vi "6733_write_waveform.vi"(8 "Error In":errorcluster, 9 "Control Task In":refnum<k21>, 10 "Waveform Task In":refnum<k21>, 11 "Inputs":T1 {"Waveform Parameters"."Degree (polynomial only)" min=1}) -> (0 "error out":errorcluster, 2 "counter task out":refnum<k21>, 3 "waveform task out":refnum<k21>)   [LabVIEW 2013]
uses:
  Control 1.ctl
  <vilib>/DAQmx/write.llb/DAQmx Write (Analog 1D DBL NChan 1Samp).vi
  <vilib>/DAQmx/write.llb/DAQmx Write (Analog 1D Wfm NChan NSamp).vi
  <vilib>/DAQmx/create/channels.llb/DAQmx Create Channel (AO-Voltage-Basic).vi
  <vilib>/DAQmx/miscellaneous.llb/DAQmx Fill In Error Info.vi
  <vilib>/Waveform/WDTOps.llb/WDT Append Waveforms DBL.vi
  <vilib>/DAQmx/configure/timing.llb/DAQmx Timing (Sample Clock).vi
  <vilib>/DAQmx/create/channels.llb/DAQmx Create Channel (CO-Pulse Generation-Frequency).vi
  <vilib>/DAQmx/configure/timing.llb/DAQmx Timing (Implicit).vi
  <vilib>/DAQmx/configure/trigger.llb/DAQmx Start Trigger (Digital Edge).vi
  <vilib>/Waveform/WDTOps.llb/WDT Scale Delta t DBL.vi
  <resource>/objmgr/daqmx.rc
panel:
  out "Total Time":dbl
  out "Sample Rate":dbl
  out "element":waveform(dbl)(graph)
  in  "index":i32
  out "Waveforms":waveform(dbl)[](array[waveform])
  out "Max Sample Rate":dbl=1000000.0
  out "# Inactive Channels":i32
  out "# Active Channels":i16
  out "Inactive Channels":tag[](array[tag])
  out "Active Channels":tag[](array[tag])
  out "Samples Written":dbl
  out "Voltage Maximum":dbl
  out "Voltage Minimum":dbl
  out "AO.PhysicalChans":tag[](array[tag])
  out "Active Device":tag
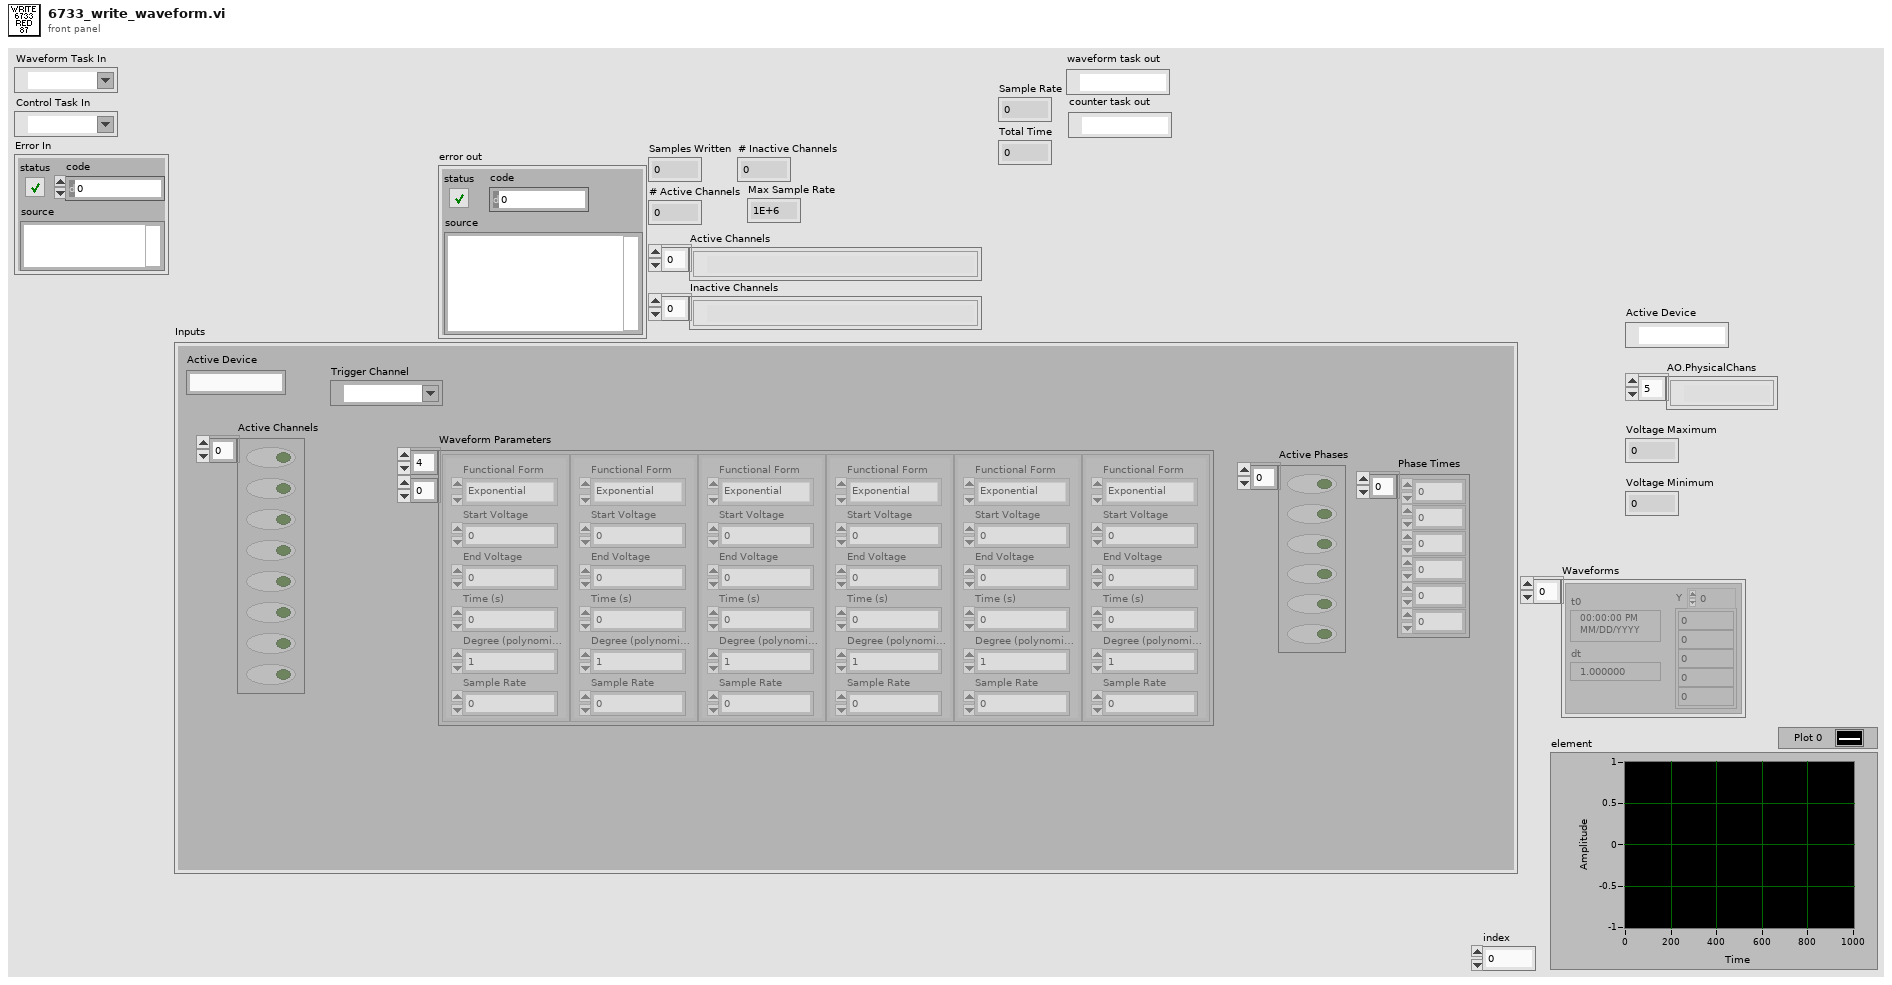
[diagram p1: front panel]
types:
  T1 = cluster{"Active Device":string, "Active Channels":bool[], "Waveform Parameters":cluster{"Functional Form":enum16{"Polynomial", "Exponential"}, "Start Voltage":dbl, "End Voltage":dbl, "Time (s)":dbl, "Degree (polynomial only)":i8, "Sample Rate":dbl}[][], "Active Phases":bool[], "Phase Times":dbl[], "Trigger Channel":tag}
  T2 = typedef "Control 1.ctl" = enum16{"Initialize", "Get Device Information", "Get Active/Inactive Channels", "Maximize Samples / Channel", "Write Waveforms", "Check for Problems", "Clear Old Tasks", "Write to cards"}
  T3 = cluster{"Functional Form":enum16{"Polynomial", "Exponential"}, "Start Voltage":dbl, "End Voltage":dbl, "Time (s)":dbl, "Degree (polynomial only)":i8, "Sample Rate":dbl}[][]
  T4 = cluster{"Functional Form":enum16{"Polynomial", "Exponential"}, "Start Voltage":dbl, "End Voltage":dbl, "Time (s)":dbl, "Degree (polynomial only)":i8, "Sample Rate":dbl}[]
  T5 = cluster{"Functional Form":enum16{"Polynomial", "Exponential"}, "Start Voltage":dbl, "End Voltage":dbl, "Time (s)":dbl, "Degree (polynomial only)":i8, "Sample Rate":dbl}
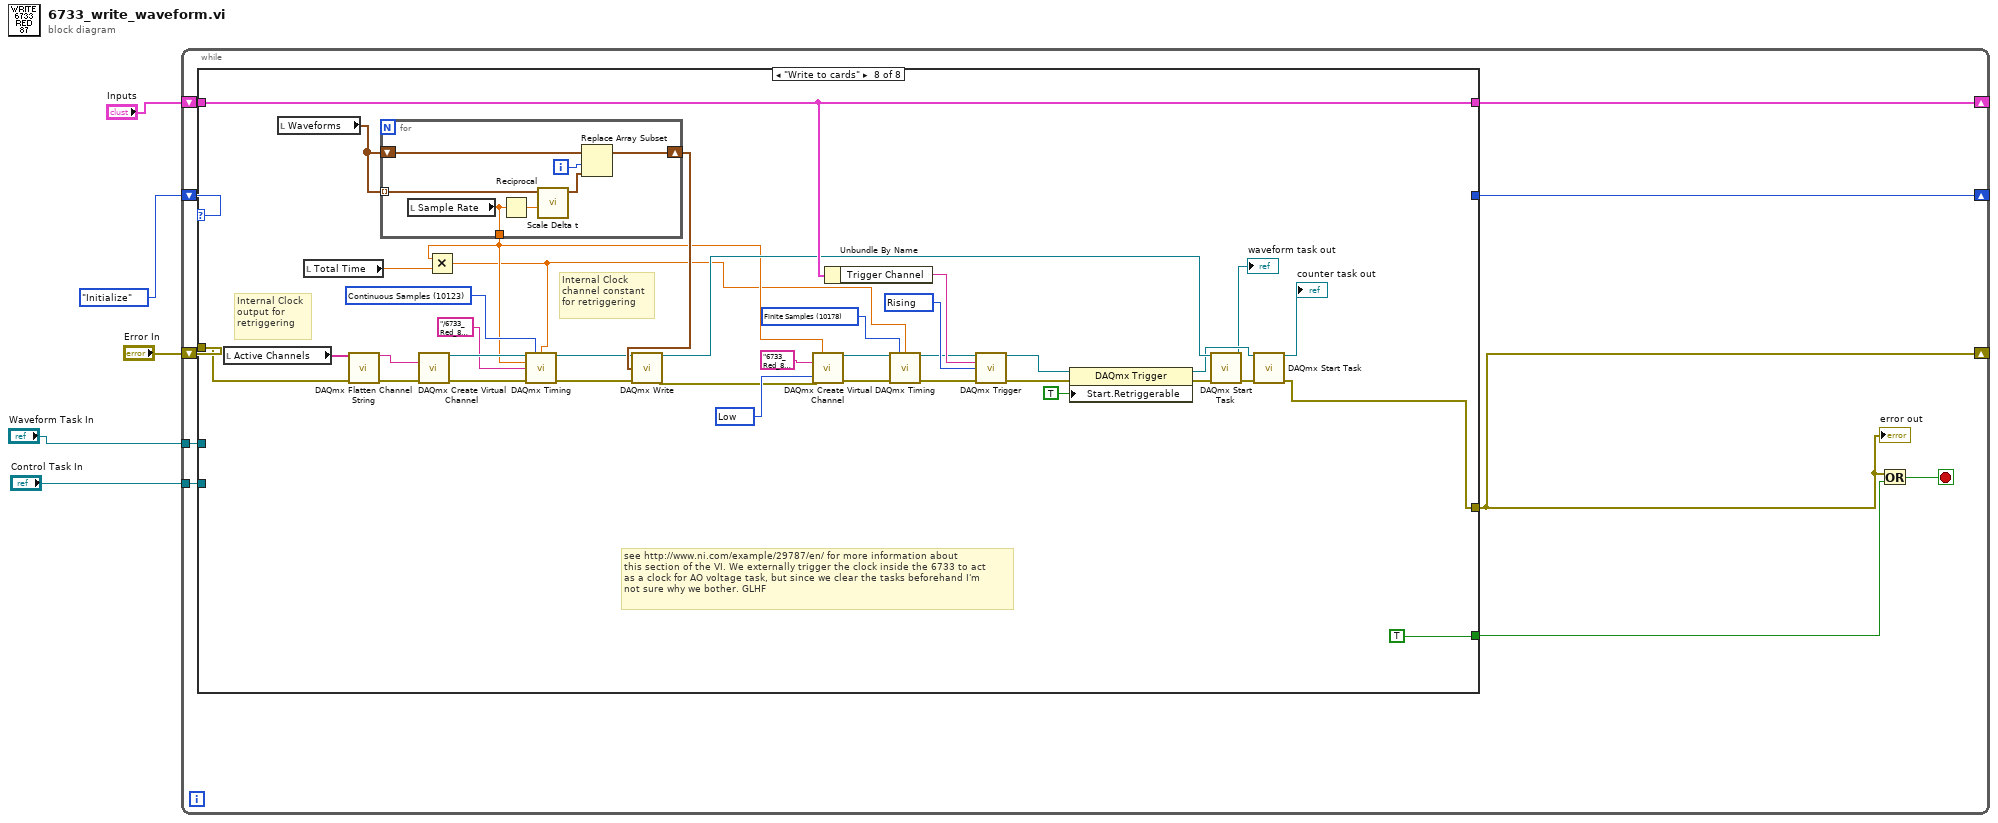
[diagram p0: block diagram]
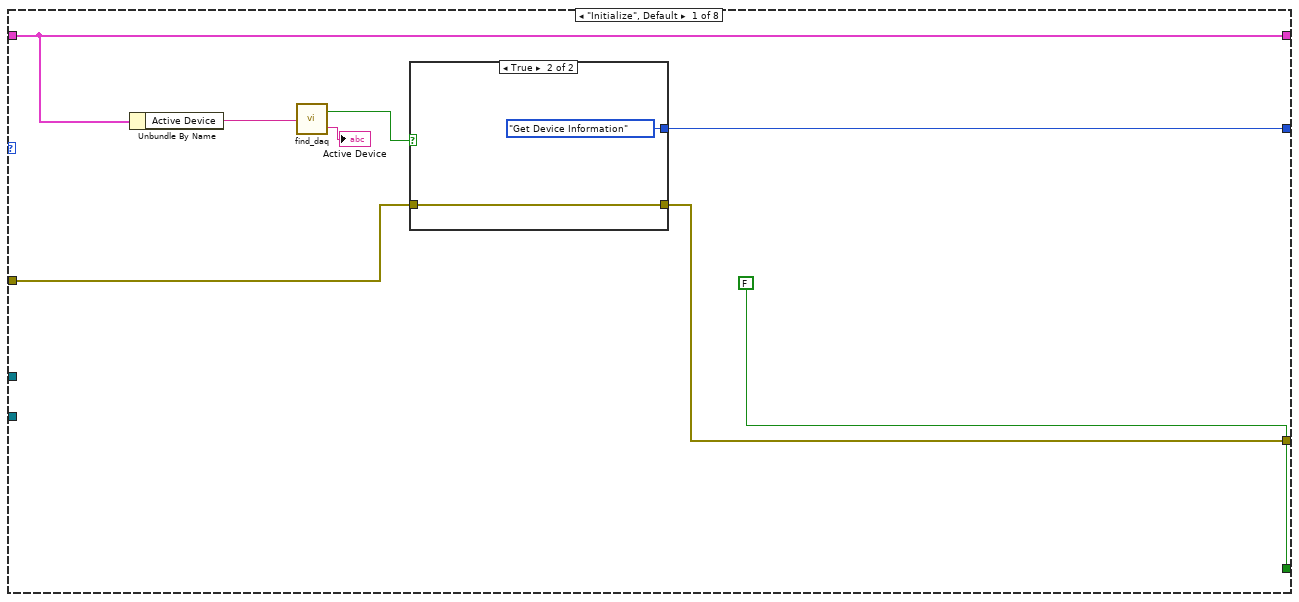
[diagram p2: hidden frame]
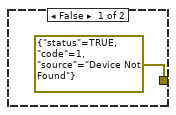
[diagram p3: hidden frame]
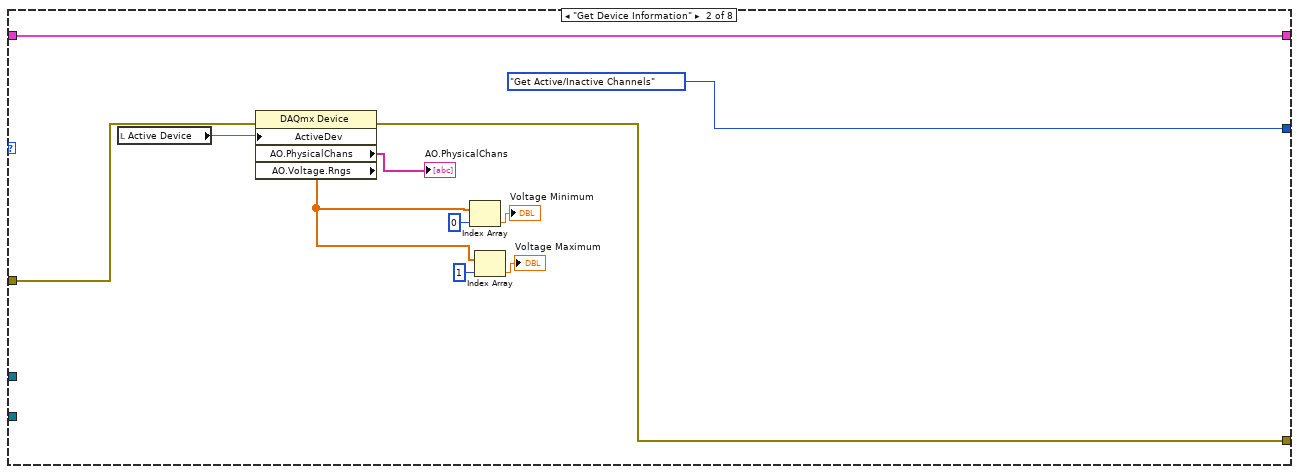
[diagram p4: hidden frame]
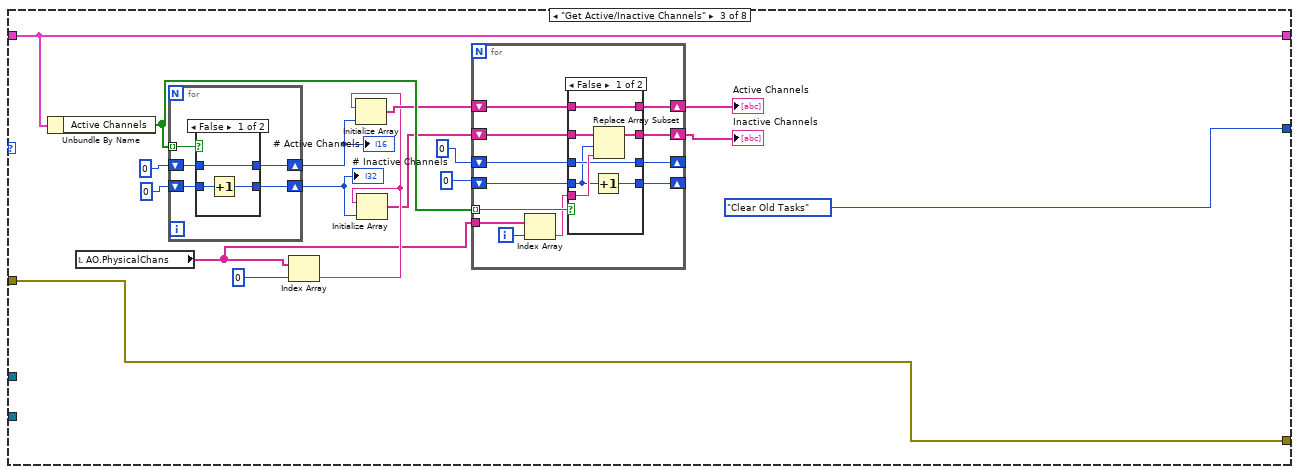
[diagram p5: hidden frame]
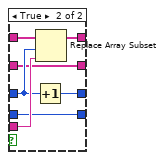
[diagram p6: hidden frame]
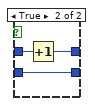
[diagram p7: hidden frame]
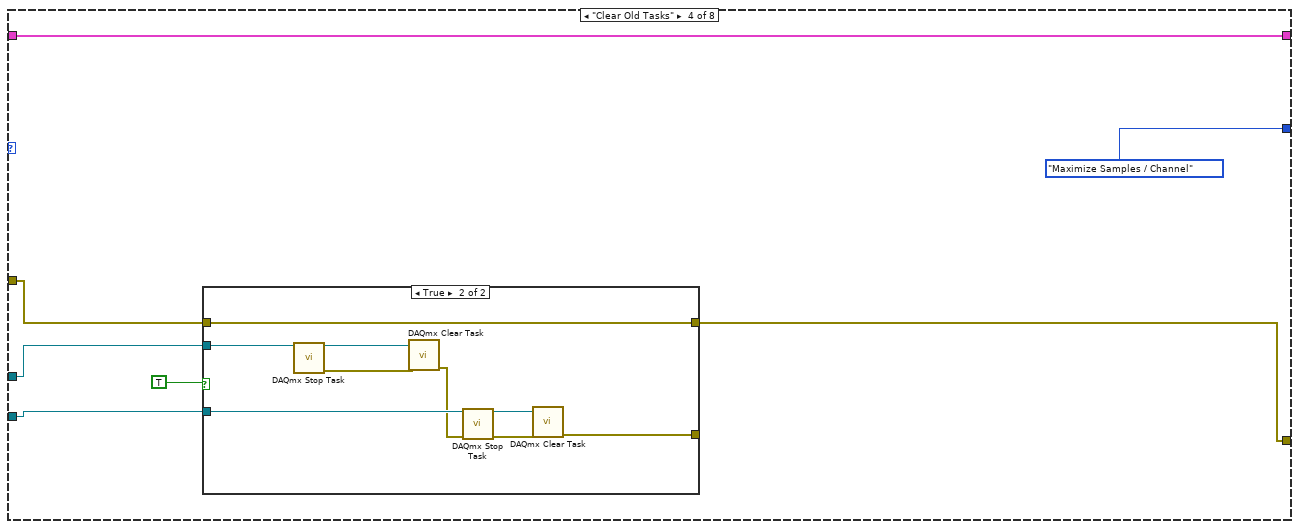
[diagram p8: hidden frame]
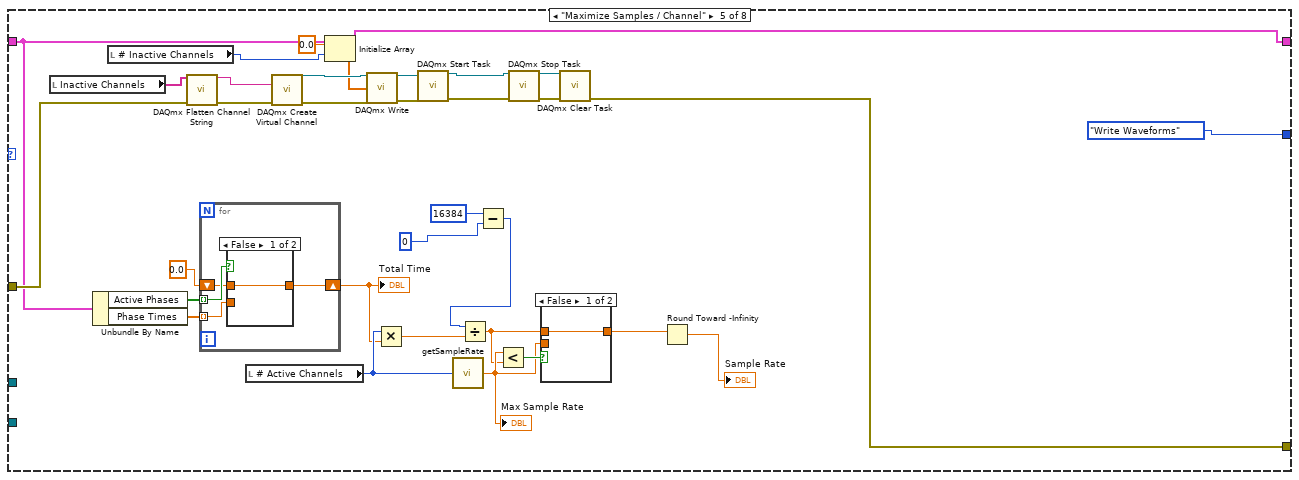
[diagram p10: hidden frame]
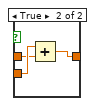
[diagram p12: hidden frame]
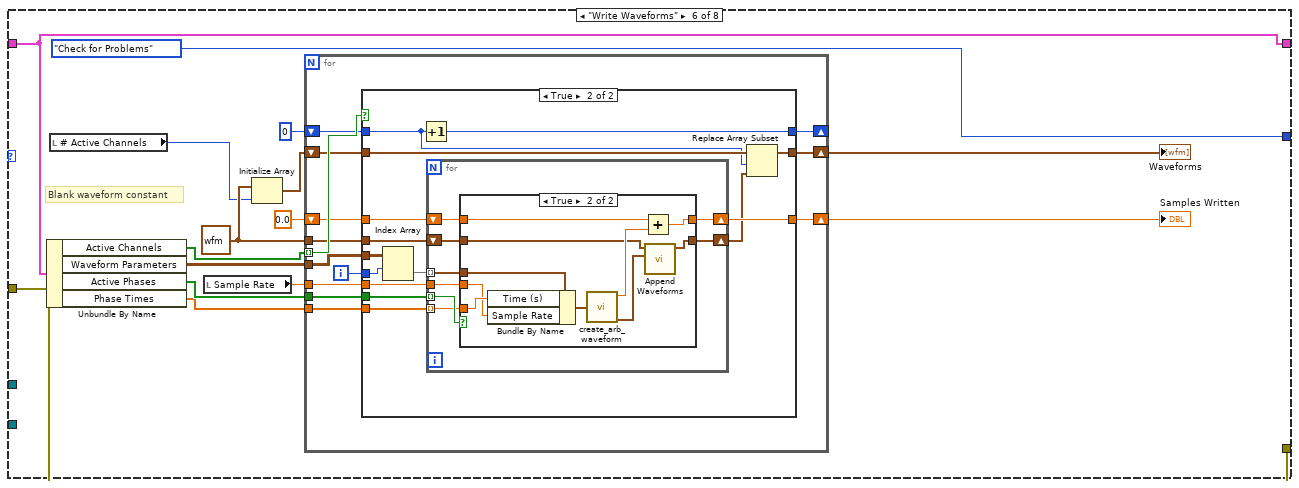
[diagram p13: hidden frame]
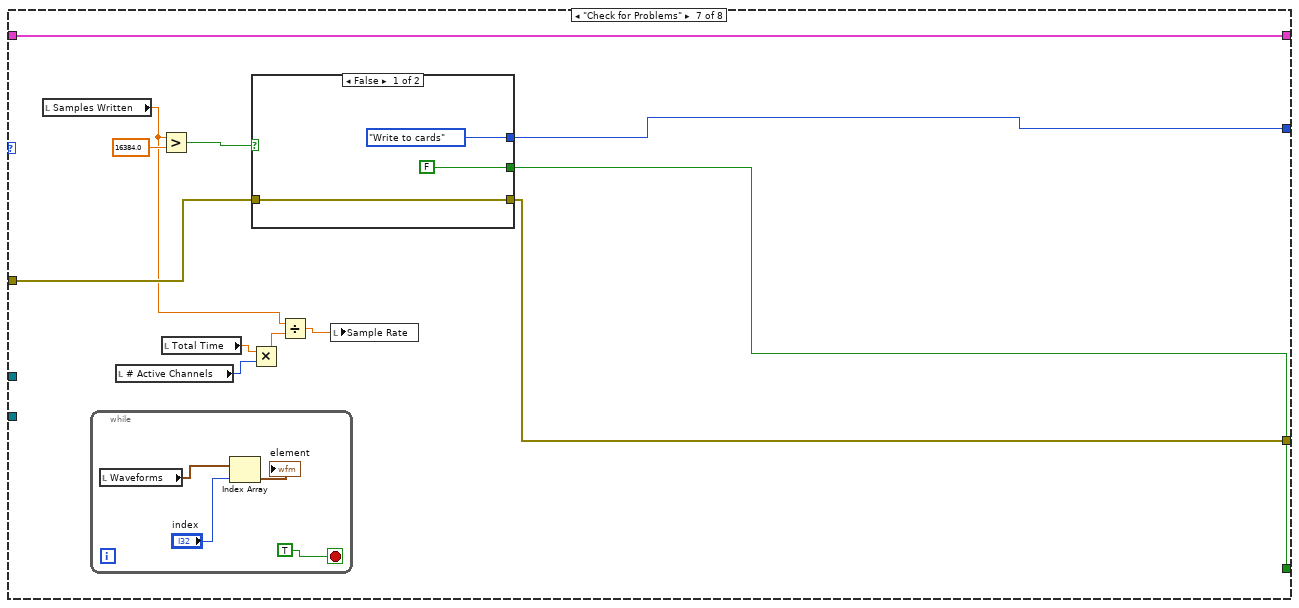
[diagram p16: hidden frame]
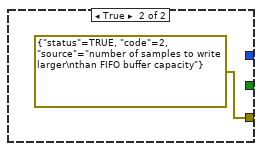
[diagram p17: hidden frame]
diagram:
  n1 = while {
    shift-right: [w11] -> _
    shift-left: "Error In" -> [w13]
    shift-right: [w12] -> _
    shift-left: Control_1."Initialize" -> [w15]
    shift-right: [w9] -> _
    shift-left: "Inputs" -> [w14]
    tunnel: "Control Task In" -> [w6]
    tunnel: "Waveform Task In" -> [w7]
    stop <- w10 stop-if-true
    n2 = case shown="\"Write to cards\"" w15 {
      tunnel: w14 -> [w17 w37 w41 w92 w123 w161 w223 w270]
      tunnel: [w20 w28 w52 w95 w127 w164 w224 w241] -> w11
      tunnel: w13 -> [w19 w36 w52 w94 w138 w164 w225 w269]
      tunnel: [w18 Control_1."Get Active/Inactive Channels" Control_1."Clear Old Tasks" Control_1."Maximize Samples / Channel" Control_1."Write Waveforms" Control_1."Check for Problems" w222 _] -> w12
      tunnel: [w17 w37 w41 w92 w123 w161 w223 w270] -> w9
      tunnel: [FALSE ("y") _ _ _ _ _ w221 TRUE ("y")] -> w8
      tunnel: w7 -> [_ _ _ w98 _ _ _ _]
      tunnel: w6 -> [_ _ _ w96 _ _ _ _]
      frame "Initialize", Default {
        n3 = Unbundle By Name(w17) -> ("Active Device"=w23:string)
        n4 = call "find_daq.vi"("Device Name"=w23) -> ("Device Present"=w21:bool, "DAQmx Device Name"=→"Active Device":tag)
        n5 = case shown="True" w21 {
          tunnel: [errorcluster {"status"=TRUE, "code"=1, "source"="Device Not Found"} ("error in (no error)") w26] -> w20
          tunnel: w19 -> [_ w26]
          tunnel: [_ Control_1."Get Device Information"] -> w18
          frame False {
          }
          frame True {
          }
        }
      }
      frame "Get Device Information" {
        n6 = local read "Active Device"() -> (w35:tag)
        n7 = property class="DAQmx Device"(error in=w36, "ActiveDev"=w35) -> (error out=w28:errorcluster, "AO.PhysicalChans"=→"AO.PhysicalChans":tag[], "AO.Voltage.Rngs"=w30:dbl[])  [unwired: 1 in, 1 out]
        n8 = Index Array(array=w30, index=0) -> (element=→"Voltage Minimum":dbl)
        n9 = Index Array(array=w30, index=1) -> (element=→"Voltage Maximum":dbl)
      }
      frame "Get Active/Inactive Channels" {
        n10 = Unbundle By Name(w41) -> ("Active Channels"=w51:bool[])
        n11 = local read "AO.PhysicalChans"() -> (w45:tag[])
        n12 = for {
          shift-right: [w85] -> w50
          shift-left: i16 0 -> [w84]
          shift-right: [w83] -> w49
          shift-left: 0 -> [w82]
          tunnel: w51 -> [w81] mode=indexing
          n13 = case shown="False" w81 {
            tunnel: [w86 w91] -> w85
            tunnel: w84 -> [w86 w90]
            tunnel: [w88 w89] -> w83
            tunnel: w82 -> [w87 w89]
            frame False {
              n14 = Increment(x=w87) -> (x+1=w88:i32)
            }
            frame True {
              n15 = Increment(x=w90) -> (x+1=w91:i16)
            }
          }
        }
        "# Active Channels" <- w50
        "# Inactive Channels" <- w49
        n16 = Index Array(array=w45, index=0) -> (element=w46:tag)
        n17 = Initialize Array(w46, w50) -> (w48:tag[])
        n18 = Initialize Array(w46, w49) -> (w44:tag[])
        n19 = for {
          tunnel: w51 -> [w66] mode=indexing
          shift-right: [w63] -> w40
          shift-left: w48 -> [w64]
          tunnel: w45 -> [w61]
          shift-right: [w59] -> w39
          shift-left: w44 -> [w60]
          shift-right: [w57] -> _
          shift-left: 0 ("index") -> [w58]
          shift-right: [w55] -> _
          shift-left: 0 ("index") -> [w56]
          i -> [w65]
          n20 = Index Array(array=w61, index=w65) -> (element=w62:tag)
          n21 = case shown="False" w66 {
            tunnel: w64 -> [w67 w80]
            tunnel: [w67 w79] -> w63
            tunnel: w62 -> [w73 w78]
            tunnel: w60 -> [w72 w74]
            tunnel: [w71 w74] -> w59
            tunnel: w58 -> [w70 w77]
            tunnel: [w70 w76] -> w57
            tunnel: w56 -> [w69 w75]
            tunnel: [w68 w75] -> w55
            frame False {
              n22 = Increment(x=w69) -> (x+1=w68:i32)
              n23 = Replace Array Subset(array=w72, new element=w73, index=w69) -> (w71:tag[])
            }
            frame True {
              n24 = Increment(x=w77) -> (x+1=w76:i32)
              n25 = Replace Array Subset(array=w80, new element=w78, index=w77) -> (w79:tag[])
            }
          }
        }
        "Active Channels" <- w40
        "Inactive Channels" <- w39
      }
      frame "Clear Old Tasks" {
        n26 = case shown="True" TRUE {
          tunnel: w98 -> [_ w108]
          tunnel: w96 -> [_ w106]
          tunnel: [w99 w104] -> w95
          tunnel: w94 -> [w99 w104]
          tunnel: [_ w100] -> _
          frame False {
          }
          frame True {
            n27 = call <vilib>:"DAQmx Stop Task.vi"("task/channels in"=w108) -> ("task out"=w107:refnum<k21>, "error out"=w103:errorcluster)  [unwired: 13 in]
            n28 = call <vilib>:"DAQmx Clear Task.vi"("task in"=w107, "error in"=w103) -> ("error out"=w102:errorcluster)  [unwired: 13 in]
            n29 = call <vilib>:"DAQmx Stop Task.vi"("task/channels in"=w106, "error in"=w102) -> ("task out"=w105:refnum<k21>, "error out"=w101:errorcluster)  [unwired: 12 in]
            n30 = call <vilib>:"DAQmx Clear Task.vi"("task in"=w105, "error in"=w101) -> ("error out"=w100:errorcluster)  [unwired: 13 in]
          }
        }
      }
      frame "Maximize Samples / Channel" {
        n31 = local read "Inactive Channels"() -> (w139:tag[])
        n32 = Unbundle By Name(w123) -> ("Active Phases"=w122:bool[], "Phase Times"=w121:dbl[])
        n33 = local read "# Inactive Channels"() -> (w132:i32)
        n34 = call <vilib>:"DAQmx Flatten Channel String.vi"("names in"=w139, "error in"=w138) -> ("names out"=w137:string, "error out"=w140:errorcluster)  [unwired: 12 in]
        n35 = for {
          tunnel: w122 -> [w146] mode=indexing
          tunnel: w121 -> [w145] mode=indexing
          shift-right: [w143] -> w114
          shift-left: 0.0 -> [w144]
          n36 = case shown="False" w146 {
            tunnel: w145 -> [_ w150]
            tunnel: w144 -> [w147 w149]
            tunnel: [w147 w148] -> w143
            frame False {
            }
            frame True {
              n37 = Add(x=w150, y=w149) -> (x+y=w148:dbl)
            }
          }
        }
        "Total Time" <- w114
        n38 = local read "# Active Channels"() -> (w115:i16)
        n39 = call-poly <vilib>:"DAQmx Create Virtual Channel.vi"("physical channels"=w137, "error in"=w140) -> ("task out"=w136:refnum<k21>, "error out"=w135:errorcluster)  [unwired: 12 in]
        n40 = Initialize Array(0.0 ("element"), w132) -> (w130:dbl[])
        n41 = call-poly <vilib>:"DAQmx Write.vi"("task/channels in"=w136, "data"=w130, "error in"=w135) -> ("task out"=w133:refnum<k21>, "error out"=w134:errorcluster)  [unwired: 10 in, 1 out]
        n42 = Multiply(x=w115, y=w114) -> (x*y=w116:dbl)
        n43 = call <vilib>:"DAQmx Start Task.vi"("task/channels in"=w133, "error in"=w134) -> ("task out"=w125:refnum<k21>, "error out"=w126:errorcluster)  [unwired: 12 in]
        n44 = call "getSampleRate.vi"("Number of active channels"=w115) -> ("Sample Rate"=w118:dbl)
        "Max Sample Rate" <- w118
        n45 = Subtract(x=16384, y=0) -> (x-y=w112:i32)
        n46 = Divide(x=w112, y=w116) -> (x/y=w117:dbl)
        n47 = Less?(x=w118, y=w117) -> (x < y?=w119:bool)
        n48 = call <vilib>:"DAQmx Stop Task.vi"("task/channels in"=w125, "error in"=w126) -> ("task out"=w129:refnum<k21>, "error out"=w128:errorcluster)  [unwired: 12 in]
        n49 = case shown="False" w119 {
          tunnel: [w141 w142] -> w110
          tunnel: w118 -> [_ w142]
          tunnel: w117 -> [w141 _]
          frame False {
          }
          frame True {
          }
        }
        n50 = call <vilib>:"DAQmx Clear Task.vi"("task in"=w129, "error in"=w128) -> ("error out"=w127:errorcluster)  [unwired: 13 in]
        n51 = Round Toward -Infinity(1:w110) -> (0:→"Sample Rate":dbl)
      }
      frame "Write Waveforms" {
        w158 = waveform(dbl) {"t0"=timestamp(0 s since 1904-01-01), "dt"=1.0, "Y"=[]}
        # "Blank waveform constant"
        n52 = Unbundle By Name(w161) -> ("Active Channels"=w153:bool[], "Waveform Parameters"=w165:T3, "Active Phases"=w159:bool[], "Phase Times"=w154:dbl[])
        n53 = local read "# Active Channels"() -> (w151:i16)
        n54 = local read "Sample Rate"() -> (w152:dbl)
        n55 = Initialize Array(w158, w151) -> (w156:waveform(dbl)[])
        n56 = for {
          tunnel: w153 -> [w178] mode=indexing
          tunnel: w165 -> [w176]
          shift-right: [w175] -> w163
          shift-left: 0.0 -> [w174]
          tunnel: w159 -> [w173]
          tunnel: w158 -> [w172]
          shift-right: [w170] -> _
          shift-left: 0 -> [w171]
          shift-right: [w168] -> w155
          shift-left: w156 -> [w169]
          tunnel: w154 -> [w167]
          tunnel: w152 -> [w166]
          i -> [w177]
          n57 = case shown="True" w178 {
            tunnel: w177 -> [_ w195]
            tunnel: w176 -> [_ w194]
            tunnel: [w181 w193] -> w175
            tunnel: w174 -> [w181 w192]
            tunnel: w173 -> [_ w190]
            tunnel: w172 -> [_ w189]
            tunnel: w171 -> [w180 w186]
            tunnel: [w180 w188] -> w170
            tunnel: w169 -> [w179 w187]
            tunnel: [w179 w184] -> w168
            tunnel: w167 -> [_ w183]
            tunnel: w166 -> [_ w182]
            frame False {
            }
            frame True {
              n58 = Index Array(array=w194, index (row)=w195) -> (element=w191:T4)  [unwired: 1 in]
              n59 = Increment(x=w186) -> (x+1=w188:i32)
              n60 = for {
                shift-right: [w203] -> w193
                shift-left: w192 -> [w202]
                tunnel: w191 -> [w201] mode=indexing
                shift-right: [w199] -> w185
                shift-left: w189 -> [w200]
                tunnel: w190 -> [w198] mode=indexing
                tunnel: w183 -> [w197] mode=indexing
                tunnel: w182 -> [w196]
                n61 = case shown="True" w198 {
                  tunnel: [w205 w214] -> w203
                  tunnel: w202 -> [w205 w213]
                  tunnel: w201 -> [_ w209]
                  tunnel: w200 -> [w204 w211]
                  tunnel: [w204 w210] -> w199
                  tunnel: w197 -> [_ w208]
                  tunnel: w196 -> [_ w206]
                  frame False {
                  }
                  frame True {
                    n62 = Bundle By Name(cluster=w209, "Time (s)"=w208, "Sample Rate"=w206) -> (w207:T5)
                    n63 = call "create_arb_waveform.vi"("Waveform Parameters"=w207) -> ("Samples to Write"=w215:dbl, "output waveform"=w212:waveform(dbl))  [unwired: 2 out]
                    n64 = Add(x=w213, y=w215) -> (x+y=w214:dbl)
                    n65 = call-poly <vilib>:"Append Waveforms.vi"("waveform B"=w212, "waveform A"=w211) -> ("waveform out"=w210:waveform(dbl))  [unwired: 8 in, 1 out]
                  }
                }
              }
              n66 = Replace Array Subset(array=w187, new element=w185, index=w186) -> (w184:waveform(dbl)[])
            }
          }
        }
        "Samples Written" <- w163
        "Waveforms" <- w155
      }
      frame "Check for Problems" {
        n67 = local read "Samples Written"() -> (w220:dbl)
        n68 = while {
          stop <- TRUE stop-if-true
          n69 = local read "Waveforms"() -> (w231:waveform(dbl)[])
          n70 = Index Array(array=w231, index="index") -> (element=→"element":waveform(dbl))
        }
        n71 = local read "# Active Channels"() -> (w217:i16)
        n72 = Greater?(x=w220, y=16384.0) -> (0:w227:bool)
        n73 = local read "Total Time"() -> (w218:dbl)
        n74 = Multiply(x=w218, y=w217) -> (x*y=w216:dbl)
        n75 = case shown="False" w227 {
          tunnel: w225 -> [w234 _]
          tunnel: [w234 errorcluster {"status"=TRUE, "code"=2, "source"="number of samples to write larger\nthan FIFO buffer capacity"} ("error in (no error)")] -> w224
          tunnel: [Control_1."Write to cards" _] -> w222
          tunnel: [FALSE ("y") _] -> w221
          frame False {
          }
          frame True {
          }
        }
        n76 = Divide(x=w220, y=w216) -> (x/y=w219:dbl)
        n77 = local write "Sample Rate"(w219) -> ()
      }
      frame "Write to cards" {
        w254 = 10280 items=["Rising"=10280, "Falling"=10171] ("edge")
        w261 = 10123 items=["Finite Samples"=10178, "Continuous Samples"=10123, "Hardware Timed Single Point"=12522] ("sample mode")
        w263 = 10178 items=["Finite Samples"=10178, "Continuous Samples"=10123, "Hardware Timed Single Point"=12522] ("sample mode")
        w266 = 10214 items=["High"=10192, "Low"=10214] ("idle state")
        # "see http://www.ni.com/example/29787/en/ for more information about\nthis section of the VI. We externally trigger the clock inside the 6733 to act\nas a clock for AO voltage task, but since we clear the tasks beforehand I'm\nnot sure why we bother. GLHF"
        # "Internal Clock\noutput for\nretriggering"
        # "Internal Clock\nchannel constant\nfor retriggering"
        n78 = local read "Active Channels"() -> (w268:tag[])
        n79 = local read "Waveforms"() -> (w271:waveform(dbl)[])
        n80 = local read "Total Time"() -> (w262:dbl)
        n81 = call <vilib>:"DAQmx Flatten Channel String.vi"("names in"=w268, "error in"=w269) -> ("names out"=w267:string, "error out"=w238:errorcluster)  [unwired: 12 in]
        n82 = for {
          tunnel: w271 -> [w279] mode=indexing
          shift-right: [w273] -> w257
          shift-left: w271 -> [w275]
          tunnel: [w274] -> w244
          i -> [w277]
          n83 = local read "Sample Rate"() -> (w274:dbl)
          n84 = Reciprocal(x=w274) -> (1/x=w278:dbl)
          n85 = call-poly <vilib>:"Scale Delta t.vi"("scale factor"=w278, "waveform in"=w279) -> ("waveform out"=w276:waveform(dbl))  [unwired: 8 in, 1 out]
          n86 = Replace Array Subset(array=w275, new element=w276, index=w277) -> (w273:waveform(dbl)[])
        }
        n87 = call-poly <vilib>:"DAQmx Create Virtual Channel.vi"("physical channels"=w267, "error in"=w238) -> ("task out"=w260:refnum<k21>, "error out"=w259:errorcluster)  [unwired: 12 in]
        n88 = Multiply(x=w244, y=w262) -> (x*y=w236:dbl)
        n89 = call-poly <vilib>:"DAQmx Timing.vi"("task/channels in"=w260, "sample mode"=w261, "samples per channel"=w236, "rate"=w244, "source"=tag "/6733_Red_87/Ctr0InternalOutput", "error in"=w259) -> ("task out"=w256:refnum<k21>, "error out"=w258:errorcluster)  [unwired: 8 in]
        n90 = call-poly <vilib>:"DAQmx Write.vi"("task/channels in"=w256, "data"=w257, "error in"=w258) -> ("task out"=w248:refnum<k21>, "error out"=w237:errorcluster)  [unwired: 10 in, 1 out]
        n91 = call-poly <vilib>:"DAQmx Create Virtual Channel.vi"("frequency"=w244, "counter"=tag "6733_Red_87/ctr0", "error in"=w237, "idle state"=w266) -> ("task out"=w265:refnum<k21>, "error out"=w264:errorcluster)  [unwired: 10 in]
        n92 = Unbundle By Name(w270) -> ("Trigger Channel"=w253:tag)
        n93 = call-poly <vilib>:"DAQmx Timing.vi"("task/channels in"=w265, "sample mode"=w263, "samples per channel"=w236, "error in"=w264) -> ("task out"=w252:refnum<k21>, "error out"=w255:errorcluster)  [unwired: 10 in]
        n94 = call-poly <vilib>:"DAQmx Trigger.vi"("task/channels in"=w252, "source"=w253, "edge"=w254, "error in"=w255) -> ("task out"=w250:refnum<k21>, "error out"=w251:errorcluster)  [unwired: 10 in]
        n95 = property class="DAQmx Trigger"(reference=w250, error in=w251, "Start.Retriggerable"=TRUE) -> (reference out=w245:refnum<k21>, error out=w247:errorcluster)
        n96 = call <vilib>:"DAQmx Start Task.vi"("task/channels in"=w248, "error in"=w247) -> ("task out"=→"waveform task out":refnum<k21>, "error out"=w246:errorcluster)  [unwired: 12 in]
        n97 = call <vilib>:"DAQmx Start Task.vi"("task/channels in"=w245, "error in"=w246) -> ("task out"=→"counter task out":refnum<k21>, "error out"=w241:errorcluster)  [unwired: 12 in]
      }
    }
    "error out" <- w11
    n98 = Or(x=w11, y=w8) -> (x .or. y?=w10:bool)
  }
